vi "SendNotification.vi"(8 "error in (no error)":errorcluster, 11 "ByRefClass in":refnum<class "ClassByRef.lvclass">) -> (0 "error out":errorcluster, 3 "ByRefClass out":refnum<class "ClassByRef.lvclass">)   [LabVIEW 2021, in "ClassUtilities.lvlib" / "ClassByRef.lvclass"]
uses:
  ClassByRef.lvclass
  ClassByRef.lvclass/ClassByRef.ctl
  GetNotifier.vi
  GetNotifier.vi/815770e3-f244-4544-877a-43bf45f14863.vi
  GetRef.vi
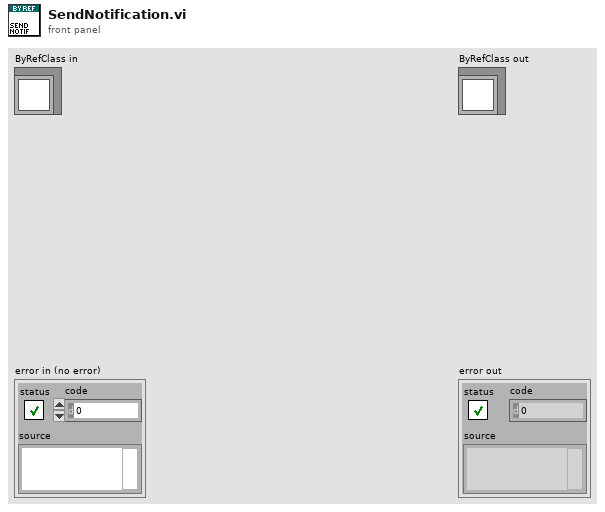
[diagram p1: front panel]
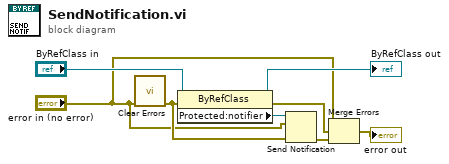
[diagram p0: block diagram]
diagram:
  n1 = call <vilib>:"Clear Errors.vi"("error in (no error)"="error in (no error)") -> ("error out"=w2:errorcluster)  [unwired: 5 in, 1 out]
  n2 = property class="ByRefClass"(reference="ByRefClass in", error in=w2) -> (reference out=→"ByRefClass out":refnum<class "ClassByRef.lvclass">, error out=w3:errorcluster, "Protected:notifier"=w8:refnum<notifier>)
  n3 = Send Notification(notification="error in (no error)", notifier=w8, error in (no error)=w2) -> (error out=w7:errorcluster)  [unwired: 1 out]
  n4 = Merge Errors("error in (no error)", w3, w7) -> (→"error out":errorcluster)
